vi "InitActor.vi"() -> (3 "Actor":refnum<class "Actor.lvclass">)   [LabVIEW 2020, in "jettl.lvlib" / "BaseActor.lvlib"]
uses:
  BaseActor.lvlib
  BaseActor/BaseActor.lvclass
  Actor/Actor.lvclass
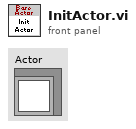
[diagram p1: front panel]
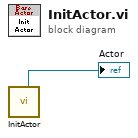
[diagram p0: block diagram]
diagram:
  n1 = call "InitActor.vi"() -> ("BaseActor"=→"Actor":refnum<class "BaseActor.lvclass">)  [unwired: 11 in]
